vi "CRYData View Legend InsDel.vi"(9 "sOption":string, 10 "Graph VI Ref":refnum<vi>, 11 "sAction":string) -> ()   [LabVIEW 2013]
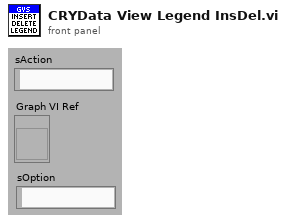
[diagram p1: front panel]
types:
  T1 = typedef "LVBoundsTypeDef.ctl" = cluster{"Width":u32, "Height":u32}
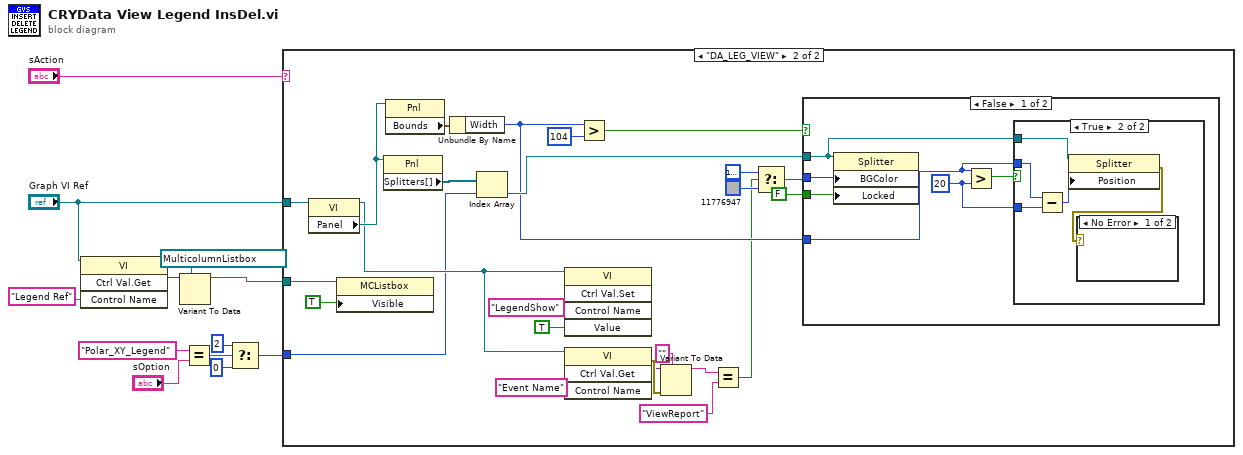
[diagram p0: block diagram]
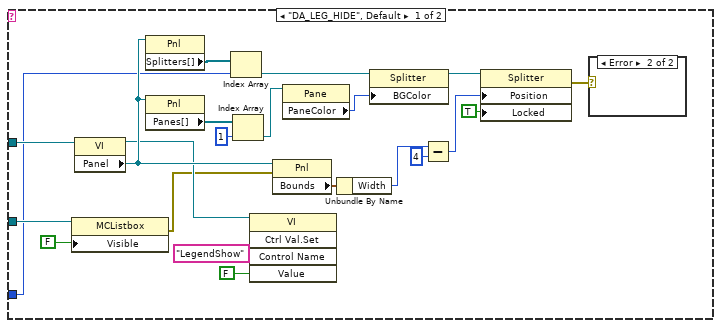
[diagram p2: hidden frame]
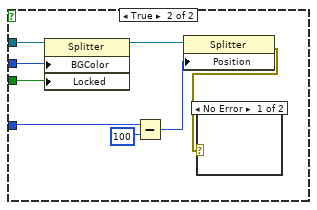
[diagram p6: hidden frame]
diagram:
  n1 = invoke class="VI" method="Ctrl Val.Get"(reference="Graph VI Ref", "Control Name"="Legend Ref") -> ("Get Control Value Variant"=w4:variant)  [unwired: 2 in, 3 out]
  n2 = Variant To Data(type=refnum<vi> refnum ("GMListbox"), Variant=w4) -> (data=w1:refnum<vi>)  [unwired: 1 in, 1 out]
  n3 = Equal?(x="Polar_XY_Legend", y="sOption") -> (x = y?=w10:bool)
  n4 = Select(t=2 ("index"), s=w10, f=0 ("index")) -> (s? t:f=w6:i32)
  n5 = case shown="\"DA_LEG_VIEW\"" "sAction" {
    tunnel: "Graph VI Ref" -> [w19 w56]
    tunnel: w1 -> [w33 w50]
    tunnel: w6 -> [w13 w35]
    frame "DA_LEG_HIDE", Default {
      n6 = property class="MCListbox"(reference=w33, "Visible"=FALSE) -> (error out=w14:errorcluster)  [unwired: 1 in, 1 out]
      n7 = property class="VI"(reference=w19) -> (reference out=w16:refnum<vi>, "Panel"=w27:refnum<vi>)  [unwired: 1 in, 1 out]
      n8 = property class="Pnl"(reference=w27) -> ("Splitters[]"=w21:refnum<vi>[])  [unwired: 1 in, 2 out]
      n9 = property class="Pnl"(reference=w27) -> ("Panes[]"=w20:refnum<vi>[])  [unwired: 1 in, 2 out]
      n10 = Index Array(array=w21, index=w13) -> (element=w22:refnum<vi>)
      n11 = Index Array(array=w20, index=1) -> (element=w24:refnum<vi>)
      n12 = invoke class="VI" method="Ctrl Val.Set"(reference=w16, "Control Name"="LegendShow", "Value"=FALSE ("Visible")) -> ()  [unwired: 2 in, 5 out]
      n13 = property class="Pnl"(reference=w27, error in=w14) -> ("Bounds"=w28:T1)  [unwired: 2 out]
      n14 = property class="Pane"(reference=w24) -> ("PaneColor"=w23:u32)  [unwired: 1 in, 2 out]
      n15 = Unbundle By Name(w28) -> ("Width"=w29:u32)
      n16 = property on="Property Node" class="Splitter"(reference=w22, "BGColor"=w23) -> (reference out=w25:refnum<vi>)  [unwired: 1 in, 1 out]
      n17 = Subtract(x=w29, y=u32 4) -> (x-y=w31:u32)
      n18 = property on="Property Node" class="Splitter"(reference=w25, "Position"=w31, "Locked"=TRUE ("Splitter Position Locked")) -> (error out=w26:errorcluster)  [unwired: 1 in, 1 out]
      n19 = case shown="Error" w26 {
        frame No Error {
        }
        frame Error {
        }
      }
    }
    frame "DA_LEG_VIEW" {
      n20 = property class="VI"(reference=w56) -> (reference out=w42:refnum<vi>, "Panel"=w58:refnum<vi>)  [unwired: 1 in, 1 out]
      n21 = property class="MCListbox"(reference=w50, "Visible"=TRUE) -> ()  [unwired: 1 in, 2 out]
      n22 = property class="Pnl"(reference=w58) -> ("Splitters[]"=w59:refnum<vi>[])  [unwired: 1 in, 2 out]
      n23 = property class="Pnl"(reference=w58) -> ("Bounds"=w57:T1)  [unwired: 1 in, 2 out]
      n24 = Unbundle By Name(w57) -> ("Width"=w51:u32)
      n25 = Index Array(array=w59, index=w35) -> (element=w53:refnum<vi>)
      n26 = invoke class="VI" method="Ctrl Val.Set"(reference=w42, "Control Name"="LegendShow", "Value"=TRUE ("Visible")) -> ()  [unwired: 2 in, 5 out]
      n27 = invoke class="VI" method="Ctrl Val.Get"(reference=w42, "Control Name"="Event Name") -> (error out=w44:errorcluster, "Get Control Value Variant"=w43:variant)  [unwired: 2 in, 2 out]
      n28 = Greater?(x=w51, y=u32 104) -> (0:w54:bool)
      n29 = Variant To Data(error in=w44, type="" ("Control Name"), Variant=w43) -> (data=w41:string)  [unwired: 1 out]
      n30 = Equal?(x=w41, y="ViewReport" ("Control Name")) -> (x = y?=w37:bool)
      n31 = Select(t=u32 16777226, s=w37, f=u32 11776947) -> (s? t:f=w38:u32)
      n32 = case shown="False" w54 {
        tunnel: w53 -> [w62 w76]
        tunnel: w38 -> [w65 w77]
        tunnel: FALSE ("Splitter Position Locked") -> [w64 w78]
        tunnel: w51 -> [w61 w74]
        frame False {
          w60 = u32 20 ("y")
          n33 = property on="Property Node" class="Splitter"(reference=w62, "BGColor"=w65, "Locked"=w64) -> ()  [unwired: 1 in, 2 out]
          n34 = Greater?(x=w61, y=w60) -> (0:w63:bool)
          n35 = case shown="True" w63 {
            tunnel: w62 -> [_ w70]
            tunnel: w61 -> [_ w69]
            tunnel: w60 -> [_ w67]
            frame False {
            }
            frame True {
              n36 = Subtract(x=w69, y=w67) -> (x-y=w68:u32)
              n37 = property on="Property Node" class="Splitter"(reference=w70, "Position"=w68) -> (error out=w66:errorcluster)  [unwired: 1 in, 1 out]
              n38 = case shown="No Error" w66 {
                frame No Error {
                }
                frame Error {
                }
              }
            }
          }
        }
        frame True {
          n39 = property on="Property Node" class="Splitter"(reference=w76, "BGColor"=w77, "Locked"=w78) -> (reference out=w72:refnum<vi>)  [unwired: 1 in, 1 out]
          n40 = Subtract(x=w74, y=u32 100) -> (x-y=w73:u32)
          n41 = property on="Property Node" class="Splitter"(reference=w72, "Position"=w73) -> (error out=w71:errorcluster)  [unwired: 1 in, 1 out]
          n42 = case shown="No Error" w71 {
            frame No Error {
            }
            frame Error {
            }
          }
        }
      }
    }
  }
